vi "_PC_Pub_ExpCondiValue_SignalRemarks.vi"(2 "error in (no error)":errorcluster, 3 "expCondiVariant":variant) -> (0 "error out":errorcluster, 1 "SignalRemarks":T1)   [LabVIEW 2018]
uses:
  <vilib>/Utility/error.llb/Error Cluster From Error Code.vi
  <vilib>/ErrorRing/Error Ring.xnode
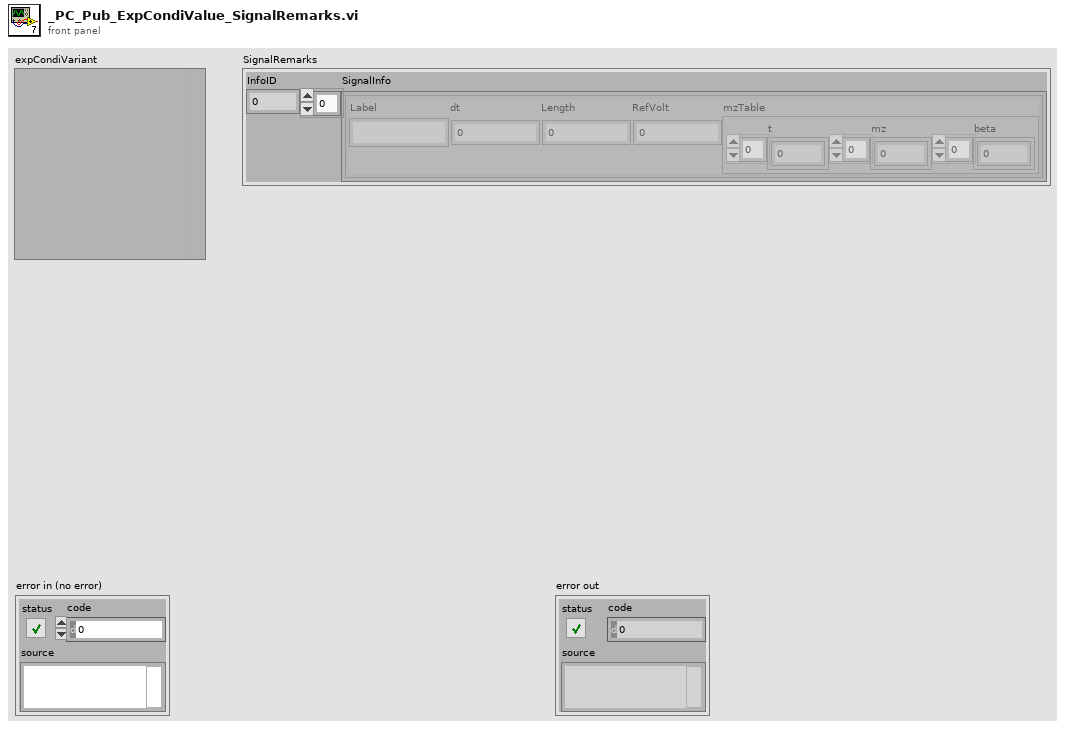
[diagram p1: front panel]
types:
  T1 = cluster{"InfoID":u64, "SignalInfo":cluster{"Label":string, "dt":dbl, "Length":u32, "RefVolt":dbl, "mzTable":cluster{"t":dbl[], "mz":dbl[], "beta":dbl[]}}[]}
  T2 = cluster{"InfoID":u64, "SignalInfo":cluster{"Label":string, "dt":dbl, "Length":u32, "RefVolt":dbl, "mzTable":cluster{"t":dbl[], "mz":dbl[], "t 2":dbl[]}}[]}
  T3 = cluster{"InfoID":u64, "SignalInfo":cluster{"Label":string, "dt":dbl, "Length":u32, "RefVolt":dbl, "mzTable":cluster{"t":dbl[], "mz":dbl[]}}[]}
  T4 = cluster{"Label":string, "dt":dbl, "Length":u32, "RefVolt":dbl, "mzTable":cluster{"t":dbl[], "mz":dbl[], "t 2":dbl[]}}
  T5 = cluster{"Label":string, "dt":dbl, "Length":u32, "RefVolt":dbl, "mzTable":cluster{"t":dbl[], "mz":dbl[]}}[]
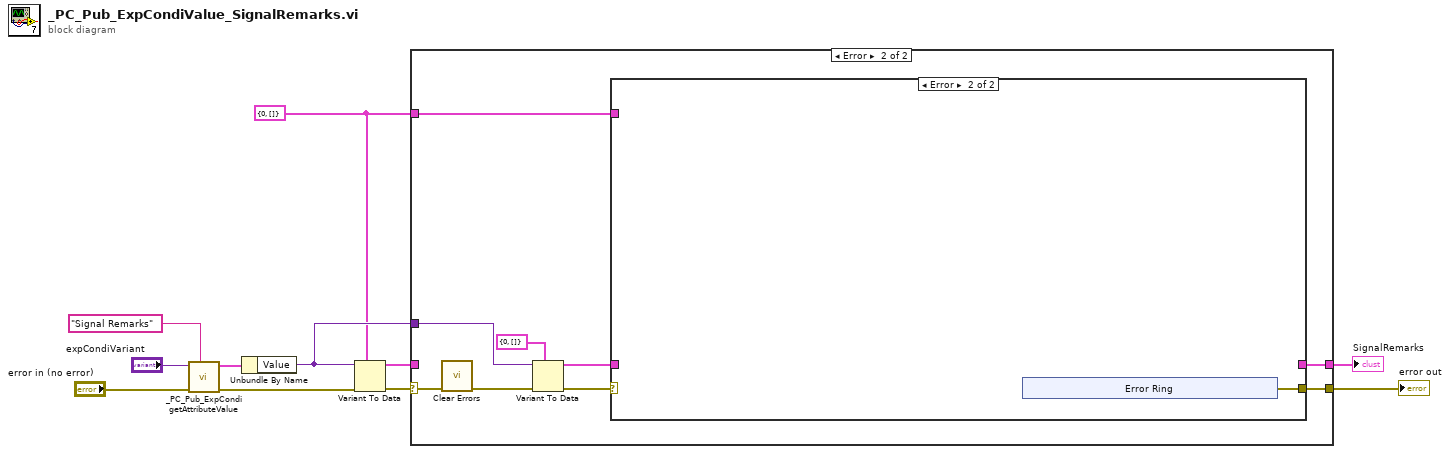
[diagram p0: block diagram]
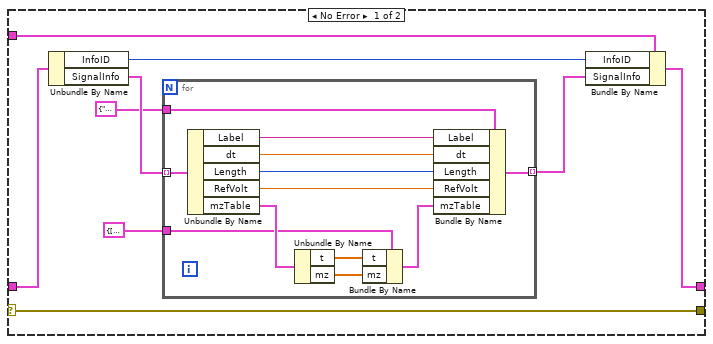
[diagram p3: hidden frame]
diagram:
  w2 = T2 {"InfoID"=0, "SignalInfo"=[]} ("SignalRemarks")
  n1 = call "_PC_Pub_ExpCondi getAttributeValue.vi"("attrName"="Signal Remarks", "error in (no error)"="error in (no error)", "expCondiVariant"="expCondiVariant") -> ("error out"=w9:errorcluster, "attrValue"=w11:cluster{"Label":string, "Value":variant})  [unwired: 7 in]
  n2 = Unbundle By Name(w11) -> ("Value"=w3:variant)
  n3 = Variant To Data(error in=w9, type=w2, Variant=w3) -> (data=w7:T2, error out=w8:errorcluster)
  n4 = case shown="Error" w8 {
    selector: w8 -> [w12 w21]
    tunnel: w7 -> [w13 _]
    tunnel: [w12 w22] -> w6
    tunnel: w3 -> [_ w19]
    tunnel: w2 -> [_ w15]
    tunnel: [w13 w14] -> w1
    frame No Error {
    }
    frame Error {
      n5 = call <vilib>:"Clear Errors.vi"("error in (no error)"=w21) -> ("error out"=w18:errorcluster)  [unwired: 5 in, 1 out]
      n6 = Variant To Data(error in=w18, type=T3 {"InfoID"=0, "SignalInfo"=[]} ("SignalRemarks"), Variant=w19) -> (data=w16:T3, error out=w17:errorcluster)
      n7 = case shown="Error" w17 {
        selector: w17 -> [w24 _]
        tunnel: [w24 w44] -> w22
        tunnel: w16 -> [w30 _]
        tunnel: w15 -> [w31 _]
        tunnel: [w23 _] -> w14
        frame No Error {
          n8 = Unbundle By Name(w30) -> ("InfoID"=w29:u64, "SignalInfo"=w28:T5)
          n9 = for {
            tunnel: w28 -> [w42] mode=indexing
            tunnel: T4 {"Label"="", "dt"=0.0, "Length"=0, "RefVolt"=0.0, "mzTable"={"t"=[], "mz"=[], "t 2"=[]}} ("Cluster") -> [w43]
            tunnel: cluster{"t":dbl[], "mz":dbl[], "t 2":dbl[]} {"t"=[], "mz"=[], "t 2"=[]} ("mzTable") -> [w36]
            tunnel: [w32] -> w25 mode=indexing
            n10 = Unbundle By Name(w42) -> ("Label"=w41:string, "dt"=w40:dbl, "Length"=w39:u32, "RefVolt"=w38:dbl, "mzTable"=w37:cluster{"t":dbl[], "mz":dbl[]})
            n11 = Unbundle By Name(w37) -> ("t"=w34:dbl[], "mz"=w33:dbl[])
            n12 = Bundle By Name(cluster=w36, "t"=w34, "mz"=w33) -> (w35:cluster{"t":dbl[], "mz":dbl[], "t 2":dbl[]})
            n13 = Bundle By Name(cluster=w43, "Label"=w41, "dt"=w40, "Length"=w39, "RefVolt"=w38, "mzTable"=w35) -> (w32:T4)
          }
          n14 = Bundle By Name(cluster=w31, "InfoID"=w29, "SignalInfo"=w25) -> (w23:T2)
        }
        frame Error {
          n15 = xnode "Error Ring"() -> ("error out"=w44:errorcluster)
        }
      }
    }
  }
  "SignalRemarks" <- w1
  "error out" <- w6
